vi "Format Build Spec Summary.vi"(8 "error in (no error)":errorcluster, 10 "VI Package Build Spec Data":T1) -> (0 "error out":errorcluster, 2 "VIPB Preview":string)   [LabVIEW 2019, in "VIPM.lvlib"]
uses:
  VIPM.lvlib
  <vilib>/JKI/VIPM API/command-line/support/VI Package Build Spec Data Cluster_vipm_api.ctl
  <vilib>/JKI/VIPM API/command-line/support/Version Info Cluster_vipm_api.ctl
  <vilib>/JKI/VIPM API/VIPM API_vipm_api.lvlib
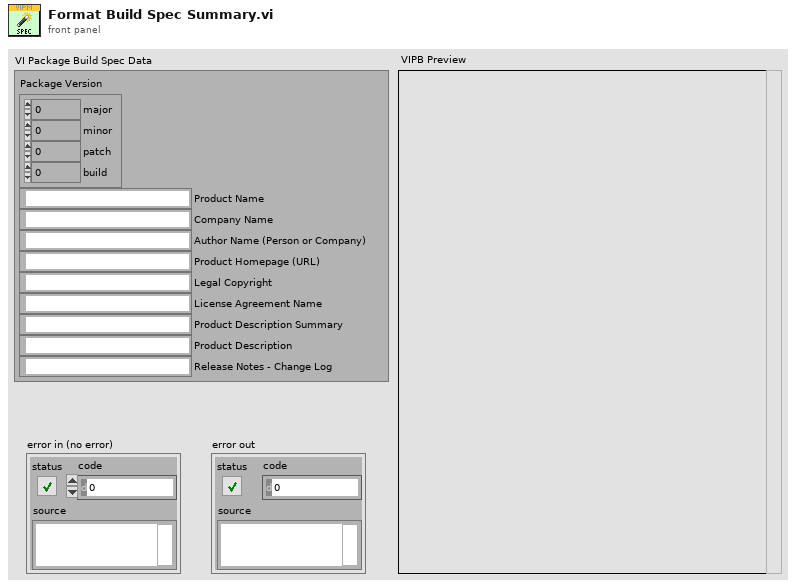
[diagram p1: front panel]
types:
  T1 = typedef "VIPM API_vipm_api.lvlib/VI Package Build Spec Data Cluster_vipm_api.ctl" = cluster{"Package Version":T2, "Product Name":string, "Company Name":string, "Author Name (Person or Company)":string, "Product Homepage (URL)":string, "Legal Copyright":string, "License Agreement Name":string, "Product Description Summary":string, "Product Description":string, "Release Notes - Change Log":string}
  T2 = typedef "VIPM API_vipm_api.lvlib/Version Info Cluster_vipm_api.ctl" = cluster{"major":u32, "minor":u32, "patch":u32, "build":u32}
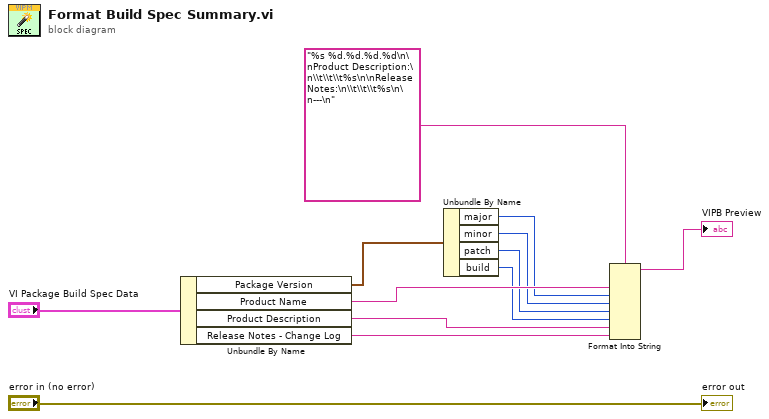
[diagram p0: block diagram]
diagram:
  n1 = Unbundle By Name("VI Package Build Spec Data") -> ("Package Version"=w12:T2, "Product Name"=w10:string, "Product Description"=w5:string, "Release Notes - Change Log"=w4:string)
  n2 = Unbundle By Name(w12) -> ("major"=w9:u32, "minor"=w8:u32, "patch"=w7:u32, "build"=w6:u32)
  n3 = Format Into String(format string="%s %d.%d.%d.%d\n\nProduct Description:\n\\t\\t\\t%s\n\nRelease Notes:\n\\t\\t\\t%s\n\n---\n", w10, w9, w8, w7, w6, w5, w4) -> (resulting string=→"VIPB Preview":string)  [unwired: 2 in, 1 out]
  "error out" <- "error in (no error)"
